vi "writeToXML.vi"(8 "error in (no error)":errorcluster, 10 "ClassLabel":string, 11 "WavefrontAbsorbOffset in":refnum<class "WavefrontAbsorbOffset.lvclass">) -> (0 "error out":errorcluster, 2 "XML out":string, 3 "WavefrontAbsorbOffset out":refnum<class "WavefrontAbsorbOffset.lvclass">)   [LabVIEW 2022 SP3, in "TCSDataDefinitions.lvlib" / "TCSCommand.lvlib" / "OffsetCommands.lvlib" / "WavefrontAbsorbOffset.lvclass"]
uses:
  WavefrontAbsorbOffset.lvclass
  AbsorbOffset/AbsorbOffset.lvclass
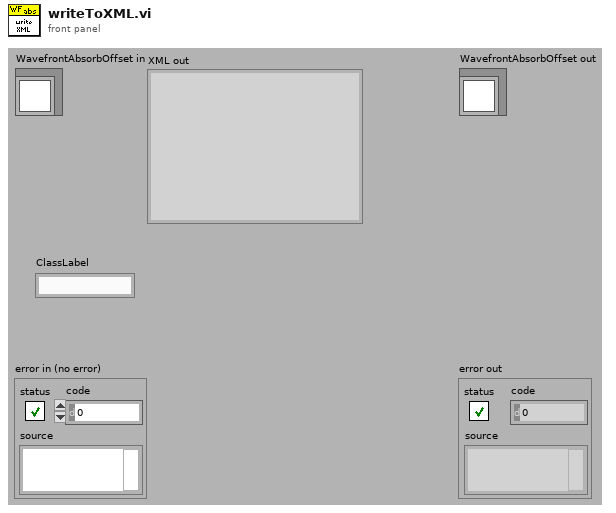
[diagram p1: front panel]
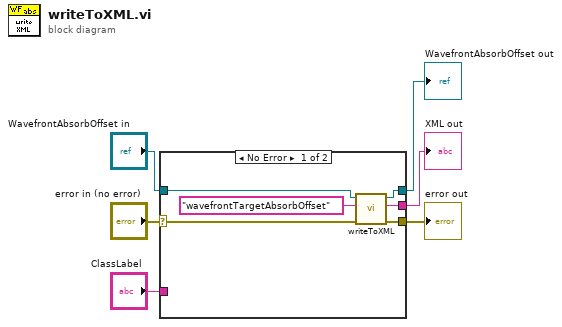
[diagram p0: block diagram]
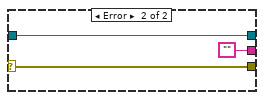
[diagram p2: hidden frame]
diagram:
  n1 = case shown="No Error" "error in (no error)" {
    selector: "error in (no error)" -> [w10 w15]
    tunnel: [w9 w15] -> w5
    tunnel: [w11 w14] -> w3
    tunnel: "WavefrontAbsorbOffset in" -> [w12 w14]
    tunnel: [w8 ""] -> w2
    tunnel: "ClassLabel" -> [_ _]
    frame No Error {
      n2 = call-parent "writeToXML.vi"("error in (no error)"=w10, "ClassLabel"="wavefrontTargetAbsorbOffset", "AbsorbOffset in"=w12) -> ("error out"=w9:errorcluster, "XML out"=w8:string, "AbsorbOffset out"=w11:refnum<class "WavefrontAbsorbOffset.lvclass">)  [unwired: 6 in]
    }
    frame Error {
    }
  }
  "error out" <- w5
  "WavefrontAbsorbOffset out" <- w3
  "XML out" <- w2
